vi "GEA2 Initialize.vi"(0 "Board Index":i32=2, 5 "Source Address":u8=228 format="%.0x", 11 "error in":errorcluster) -> (4 "GEA2 Reference Out":refnum<k24>, 8 "Board ID":string, 15 "error out":errorcluster={"status"=TRUE, "code"=1172, "source"="Invoke Node Error calling method GeaCommunication.GeaNode.RegisterAddress, (System.ArgumentNullException: Key cannot be null.\r\nParameter name: key) <append><b>System.ArgumentNullException</b> in GEA2 Initialize.vi->ReadERD's_and_Faults.vi"})   [LabVIEW 2023]
doc: "This VI uses .NET DLLs to initialize a GEA2 connection over USB. The output is a reference to the newly opened GEA2 connection."
uses:
  D:/Common/LabVIEW GEA2 Toolkit/source/GEA3 DLL Source/GeaCommunication.dll
  source/GEA3 DLL Source/GeaCommunication.dll
panel:
  in  "IPC?":bool
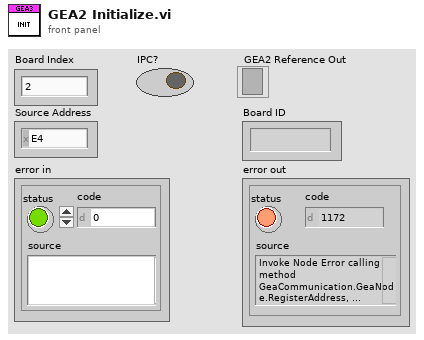
[diagram p1: front panel]
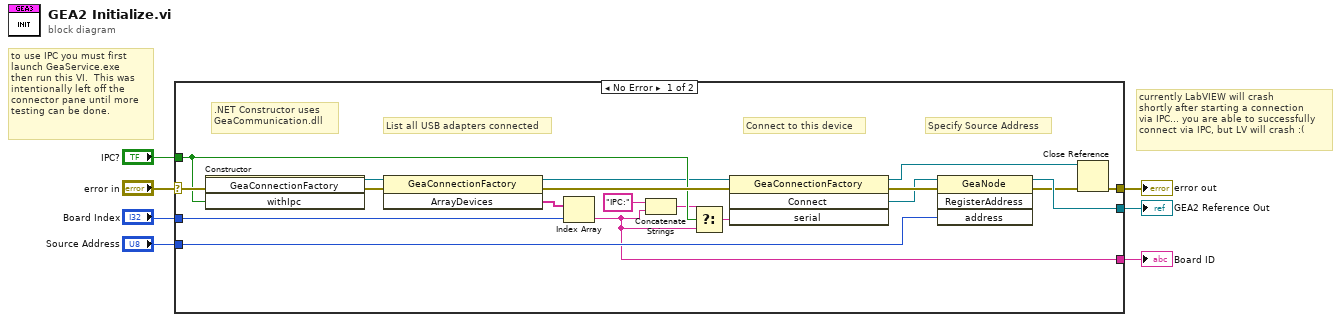
[diagram p0: block diagram]
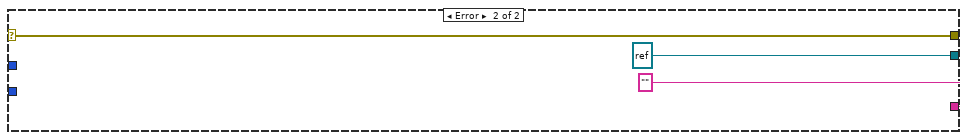
[diagram p2: hidden frame]
diagram:
  # "currently LabVIEW will crash\nshortly after starting a connection\nvia IPC... you are able to successfully\nconnect via IPC, but LV will crash :("
  # "to use IPC you must first\nlaunch GeaService.exe\nthen run this VI.  This was\nintentionally left off the\nconnector pane until more\ntesting can be done."
  n1 = case shown="No Error" "error in" {
    selector: "error in" -> [w21 w29]
    tunnel: "Board Index" -> [w18 _]
    tunnel: [w16 w29] -> w7
    tunnel: [w24 refnum<k24> refnum ("Connect")] -> w5
    tunnel: "Source Address" -> [w22 _]
    tunnel: [w12 "" ("get_Item")] -> w2
    tunnel: "IPC?" -> [w14 _]
    frame No Error {
      # "Specify Source Address"
      # "Connect to this device"
      # "List all USB adapters connected"
      # ".NET Constructor uses\nGeaCommunication.dll"
      n2 = constructor class="GeaConnectionFactory"(error in=w21, "withIpc"=w14) -> (reference out=w15:refnum<k24>, error out=w20:errorcluster)  [unwired: 2 in, 2 out]
      n3 = invoke class="GeaConnectionFactory" method="ArrayDevices"(reference=w15, error in=w20) -> (reference out=w8:refnum<k24>, error out=w17:errorcluster, "ArrayDevices"=w10:string[])  [unwired: 1 in]
      n4 = Index Array(array=w10, index=w18) -> (element=w12:string)
      n5 = Concatenate Strings("IPC:" ("string"), w12) -> (w11:string)
      n6 = Select(t=w11, s=w14, f=w12) -> (s? t:f=w9:string)
      n7 = invoke class="GeaConnectionFactory" method="Connect"(reference=w8, error in=w17, "serial"=w9) -> (reference out=w25:refnum<k24>, error out=w26:errorcluster, "Connect"=w19:refnum<k24>)  [unwired: 1 in, 1 out]
      n8 = invoke class="GeaNode" method="RegisterAddress"(reference=w19, error in=w26, "address"=w22) -> (reference out=w24:refnum<k24>, error out=w23:errorcluster)  [unwired: 1 in, 2 out]
      n9 = Close Reference(reference=w25, error in (no error)=w23) -> (error out=w16:errorcluster)
    }
    frame Error {
    }
  }
  "error out" <- w7
  "GEA2 Reference Out" <- w5
  "Board ID" <- w2
